vi "SP Get De-Embed Data From Run Data.vi"(8 "error in (no error)":errorcluster, 10 "Run Waveforms":waveform(dbl)[](array[waveform]), 11 "File Information":T2) -> (0 "error out":errorcluster, 1 "SP Data":T1, 3 "Valid?":bool)   [LabVIEW 2011]
uses:
  server/TDMS/TDMS File.ctl
  server/TDMS/TDMS Run.ctl
  server/TDMS/TDMS Channel (Sxx).ctl
  server/database/Fields/Field Record.ctl
  server/database/Fields/Field DataTypes.ctl
  server/database/Fields/Field NextItem.ctl
  TypeDefs/SP Data.ctl
  TypeDefs/SP Parameter.ctl
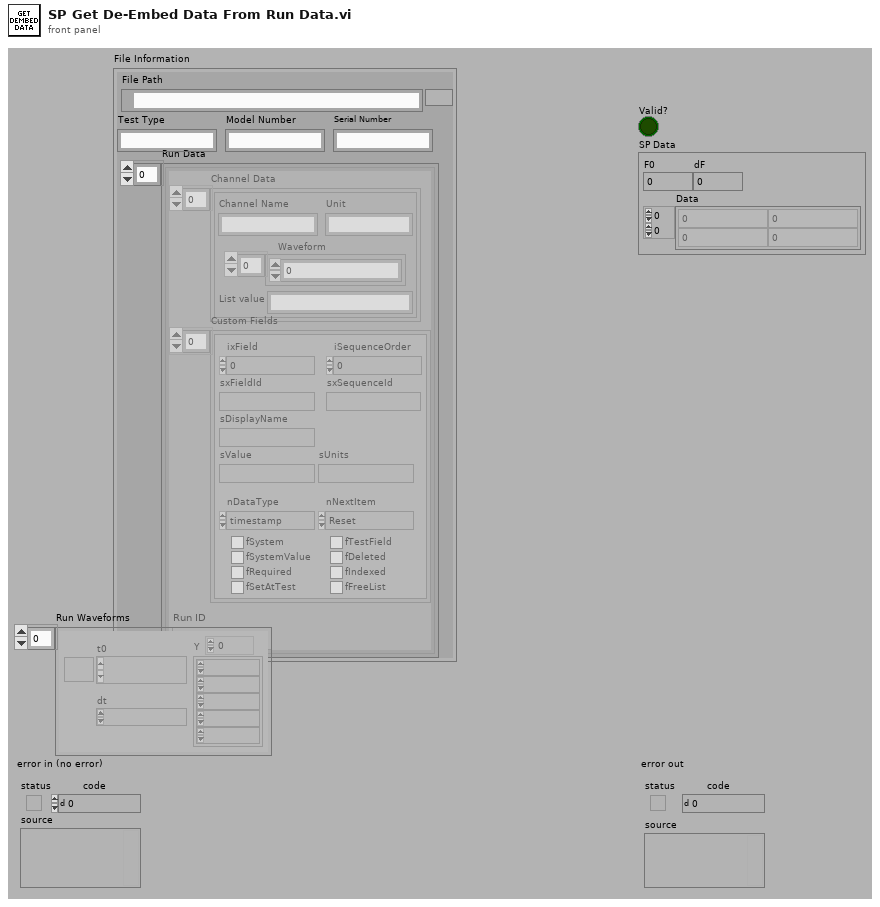
[diagram p1: front panel]
types:
  T1 = typedef "SP Data.ctl" = cluster{"F0":dbl, "dF":dbl, "Data":cdb[][]}
  T2 = typedef "TDMS File.ctl" = cluster{"File Path":path, "Run Data":T3[], "Serial Number":string, "Model Number":string, "Test Type":string}
  T3 = typedef "TDMS Run.ctl" = cluster{"Channel Data":T4[], "Custom Fields":T5[], "Run ID":string}
  T4 = typedef "TDMS Channel (Sxx).ctl" = cluster{"Channel Name":string, "Waveform":dbl[], "Unit":string, "List value":string}
  T5 = typedef "Field Record.ctl" = cluster{"ixField":i32, "iSequenceOrder":i32, "sxFieldId":string, "sxSequenceId":string, "sDisplayName":string, "sValue":string, "sUnits":string, "nDataType":T6, "nNextItem":T7, "fSystem":bool, "fSystemValue":bool, "fRequired":bool, "fSetAtTest":bool, "fTestField":bool, "fDeleted":bool, "fIndexed":bool, "fFreeList":bool}
  T6 = typedef "Field DataTypes.ctl" = enum32{"text", "numeric", "list", "timestamp", "boolean"}
  T7 = typedef "Field NextItem.ctl" = enum32{"Reset", "Retain", "Auto-Increment"}
  T8 = typedef "SP Parameter.ctl" = cluster{"Stimulus Port":i8, "Response Port":i8}
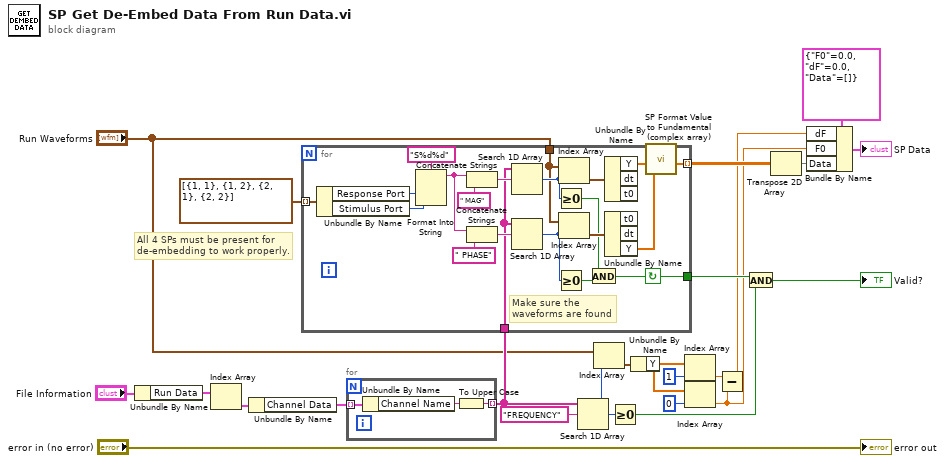
[diagram p0: block diagram]
diagram:
  # "All 4 SPs must be present for\nde-embedding to work properly."
  n1 = Unbundle By Name("File Information") -> ("Run Data"=w22:T3[])
  n2 = Index Array(array=w22) -> (element=w23:T3)  [unwired: 1 in]
  n3 = Unbundle By Name(w23) -> ("Channel Data"=w20:T4[])
  n4 = for {
    tunnel: w20 -> [w27] mode=indexing
    tunnel: [w25] -> w14 mode=indexing
    n5 = Unbundle By Name(w27) -> ("Channel Name"=w26:string)
    n6 = To Upper Case(1:w26) -> (0:w25:string)
  }
  n7 = for {
    tunnel: T8[] [{"Stimulus Port"=1, "Response Port"=1}, {"Stimulus Port"=1, "Response Port"=2}, {"Stimulus Port"=2, "Response Port"=1}, {"Stimulus Port"=2, "Response Port"=2}] -> [w45] mode=indexing
    tunnel: w14 -> [w39]
    tunnel: [w31] -> w12
    tunnel: "Run Waveforms" -> [w36]
    tunnel: [w32] -> w17 mode=indexing
    stop <- w31 continue-if-true
    # "Make sure the\nwaveforms are found"
    n8 = Unbundle By Name(w45) -> ("Response Port"=w47:i8, "Stimulus Port"=w46:i8)
    n9 = Format Into String(format string="S%d%d", w47, w46) -> (resulting string=w42:string)  [unwired: 2 in, 1 out]
    n10 = Concatenate Strings(w42, " MAG" ("format string")) -> (w44:string)
    n11 = Concatenate Strings(w42, " PHASE" ("format string")) -> (w40:string)
    n12 = Search 1D Array(1D array=w39, element=w44) -> (index of element=w38:i32)  [unwired: 1 out]
    n13 = Search 1D Array(1D array=w39, element=w40) -> (index of element=w37:i32)  [unwired: 1 out]
    n14 = Greater Or Equal To 0?(x=w38) -> (x >= 0?=w29:bool)
    n15 = Greater Or Equal To 0?(x=w37) -> (x >= 0?=w28:bool)
    n16 = Index Array(array=w36, index=w38) -> (element=w30:waveform(dbl))
    n17 = Index Array(array=w36, index=w37) -> (element=w35:waveform(dbl))
    n18 = And(x=w29, y=w28) -> (x .and. y?=w31:bool)
    n19 = Unbundle By Name(w30) -> ("Y"=w33:dbl[])  [unwired: 2 out]
    n20 = Unbundle By Name(w35) -> ("Y"=w34:dbl[])  [unwired: 2 out]
    n21 = call "SP Format Value to Fundamental (complex array).vi"("Display Values (Phase)"=w34, "Display Values (Mag)"=w33) -> ("Stored Values"=w32:cdb[])  [unwired: 5 out]
  }
  n22 = Search 1D Array(1D array=w14, element="FREQUENCY") -> (index of element=w8:i32)  [unwired: 1 out]
  n23 = Index Array(array="Run Waveforms", index=w8) -> (element=w7:waveform(dbl))
  n24 = Greater Or Equal To 0?(x=w8) -> (x >= 0?=w11:bool)
  n25 = Unbundle By Name(w7) -> ("Y"=w6:dbl[])
  n26 = Index Array(array=w6, index=1) -> (element=w3:dbl)
  n27 = Index Array(array=w6, index=0) -> (element=w1:dbl)
  n28 = Subtract(x=w3, y=w1) -> (x-y=w2:dbl)
  n29 = And(x=w12, y=w11) -> (x .and. y?=→"Valid?":bool)
  n30 = Transpose 2D Array(2D array=w17) -> (transposed array=w15:cdb[][])
  n31 = Bundle By Name(cluster=T1 {"F0"=0.0, "dF"=0.0, "Data"=[]} ("SP Data"), "dF"=w2, "F0"=w1, "Data"=w15) -> (→"SP Data":T1)
  "error out" <- "error in (no error)"
